vi "Stability Timer.vi"(0 "CommandCluster":T1, 2 "Mode":enum16{"Init", "Run"}(ring)=enum."Run", 7 "Stable":bool, 9 "Stable 2":bool, 11 "Stable 3":bool, 12 "time":refnum<vi>, 13 "time 2":refnum<vi>, 14 "time 3":refnum<vi>) -> (4 "GraphSig":bool, 15 "Stabilized?":bool)   [LabVIEW 2013]
uses:
  TypeDef/Command Cluster.ctl
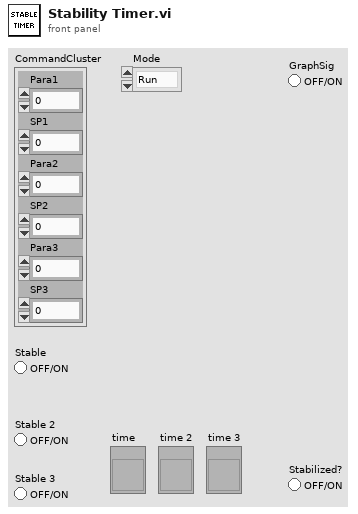
[diagram p1: front panel]
types:
  T1 = typedef "Command Cluster.ctl" = cluster{"Para1":i32, "SP1":dbl, "Para2":i32, "SP2":dbl, "Para3":i32, "SP3":dbl}
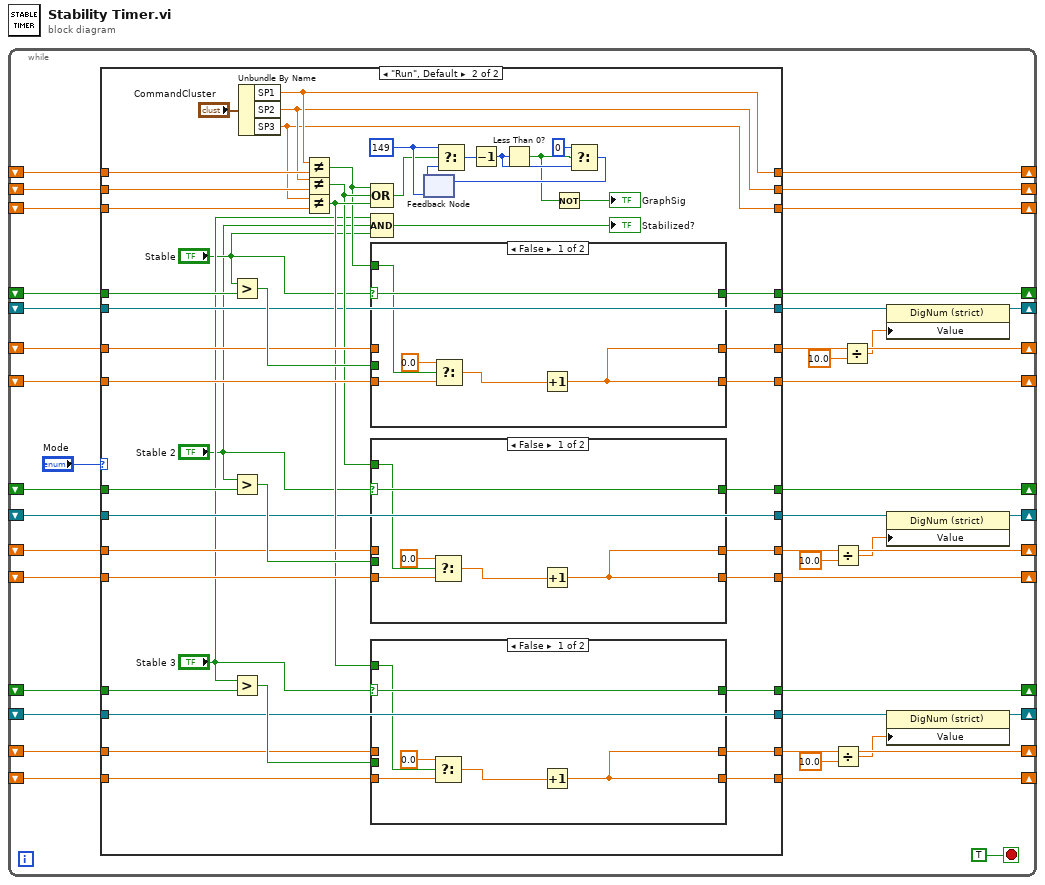
[diagram p0: block diagram]
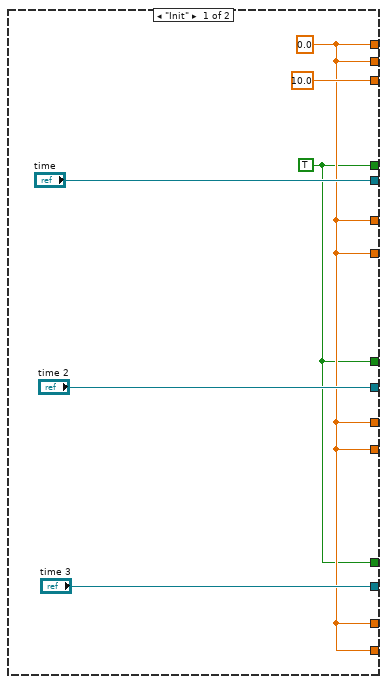
[diagram p2: hidden frame]
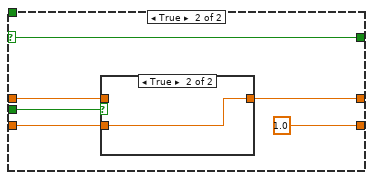
[diagram p3: hidden frame]
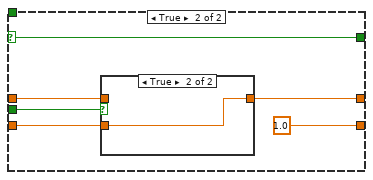
[diagram p5: hidden frame]
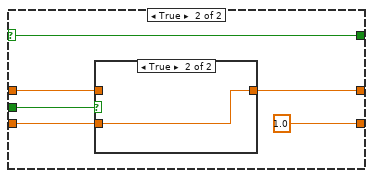
[diagram p7: hidden frame]
diagram:
  n1 = while {
    shift-right: [w40] -> _
    shift-left: _ -> [w37]
    shift-right: [w38] -> _
    shift-left: _ -> [w39]
    shift-right: [w36] -> _
    shift-left: _ -> [w35]
    shift-right: [w34] -> _
    shift-left: _ -> [w33]
    shift-right: [w10] -> _
    shift-left: _ -> [w32]
    shift-right: [w11] -> _
    shift-left: _ -> [w31]
    shift-right: [w28] -> _
    shift-left: _ -> [w29]
    shift-right: [w27] -> _
    shift-left: _ -> [w30]
    shift-right: [w26] -> _
    shift-left: _ -> [w21]
    shift-right: [w12] -> _
    shift-left: _ -> [w22]
    shift-right: [w25] -> _
    shift-left: _ -> [w20]
    shift-right: [w23] -> _
    shift-left: _ -> [w24]
    shift-right: [w5] -> _
    shift-left: _ -> [w16]
    shift-right: [w4] -> _
    shift-left: _ -> [w17]
    shift-right: [w8] -> _
    shift-left: _ -> [w18]
    stop <- TRUE stop-if-true
    n2 = case shown="\"Run\", Default" "Mode" {
      tunnel: [w42 w94] -> w40
      tunnel: w39 -> [_ w93]
      tunnel: [w43 w92] -> w38
      tunnel: w37 -> [_ w91]
      tunnel: [w42 w88] -> w36
      tunnel: w35 -> [_ w87]
      tunnel: [w43 w86] -> w34
      tunnel: w33 -> [_ w85]
      tunnel: [w43 w84] -> w10
      tunnel: w32 -> [_ w83]
      tunnel: [w43 w82] -> w11
      tunnel: w31 -> [_ w81]
      tunnel: w30 -> [_ w79]
      tunnel: w29 -> [_ w78]
      tunnel: [w43 w77] -> w28
      tunnel: [w43 w76] -> w27
      tunnel: [w43 w75] -> w12
      tunnel: [w43 w74] -> w26
      tunnel: [w42 w73] -> w25
      tunnel: w24 -> [_ w72]
      tunnel: [10.0 ("SP3") w71] -> w23
      tunnel: w22 -> [_ w69]
      tunnel: w21 -> [_ w68]
      tunnel: w20 -> [_ w67]
      tunnel: ["time" w63] -> w9
      tunnel: ["time 2" w62] -> w6
      tunnel: ["time 3" w61] -> w7
      tunnel: w18 -> [_ w63]
      tunnel: w17 -> [_ w62]
      tunnel: w16 -> [_ w61]
      frame "Init" {
        w42 = TRUE
        w43 = 0.0 ("SP1")
      }
      frame "Run", Default {
        w55 = 149
        n3 = Greater?(x="Stable", y=w91) -> (0:w90:bool)
        n4 = Greater?(x="Stable 2", y=w87) -> (0:w89:bool)
        n5 = Greater?(x="Stable 3", y=w67) -> (0:w70:bool)
        n6 = Unbundle By Name("CommandCluster") -> ("SP1"=w77:dbl, "SP2"=w76:dbl, "SP3"=w71:dbl)
        n7 = Not Equal?(x=w77, y=w78) -> (x != y?=w64:bool)
        n8 = Not Equal?(x=w76, y=w79) -> (x != y?=w65:bool)
        n9 = Not Equal?(x=w71, y=w72) -> (x != y?=w66:bool)
        n10 = Compound Arithmetic op=OR(w64, w65, w66) -> (w54:bool)
        n11 = Compound Arithmetic op=AND("Stable 3", "Stable 2", "Stable") -> (→"Stabilized?":bool)
        n12 = case shown="False" "Stable" {
          selector: "Stable" -> [w128 w133]
          tunnel: [w128 w133] -> w94
          tunnel: w93 -> [w125 w131]
          tunnel: [w127 1.0 ("y")] -> w92
          tunnel: w90 -> [_ w132]
          tunnel: [w127 w130] -> w84
          tunnel: w83 -> [_ w129]
          tunnel: w64 -> [w126 _]
          frame False {
            n13 = Select(t=0.0, s=w126, f=w125) -> (s? t:f=w124:dbl)
            n14 = Increment(x=w124) -> (x+1=w127:dbl)
          }
          frame True {
            n15 = case shown="True" w132 {
              tunnel: w131 -> [_ w136]
              tunnel: [w135 w136] -> w130
              tunnel: w129 -> [w135 _]
              frame False {
              }
              frame True {
              }
            }
          }
        }
        n16 = case shown="False" "Stable 2" {
          selector: "Stable 2" -> [w114 w119]
          tunnel: [w114 w119] -> w88
          tunnel: w85 -> [w111 w117]
          tunnel: [w113 1.0 ("y")] -> w86
          tunnel: w89 -> [_ w118]
          tunnel: [w113 w116] -> w82
          tunnel: w81 -> [_ w115]
          tunnel: w65 -> [w112 _]
          frame False {
            n17 = Select(t=0.0, s=w112, f=w111) -> (s? t:f=w110:dbl)
            n18 = Increment(x=w110) -> (x+1=w113:dbl)
          }
          frame True {
            n19 = case shown="True" w118 {
              tunnel: w117 -> [_ w122]
              tunnel: [w121 w122] -> w116
              tunnel: w115 -> [w121 _]
              frame False {
              }
              frame True {
              }
            }
          }
        }
        n20 = case shown="False" "Stable 3" {
          selector: "Stable 3" -> [w100 w105]
          tunnel: [w100 w105] -> w73
          tunnel: w68 -> [w97 w103]
          tunnel: [w99 1.0 ("y")] -> w74
          tunnel: w70 -> [_ w104]
          tunnel: [w99 w102] -> w75
          tunnel: w69 -> [_ w101]
          tunnel: w66 -> [w98 _]
          frame False {
            n21 = Select(t=0.0, s=w98, f=w97) -> (s? t:f=w96:dbl)
            n22 = Increment(x=w96) -> (x+1=w99:dbl)
          }
          frame True {
            n23 = case shown="True" w104 {
              tunnel: w103 -> [_ w108]
              tunnel: [w107 w108] -> w102
              tunnel: w101 -> [w107 _]
              frame False {
              }
              frame True {
              }
            }
          }
        }
        n24 = feedback #1(w55) -> (w56:i32)
        n25 = Select(t=w55, s=w54, f=w56) -> (s? t:f=w60:i32)
        n26 = Decrement(x=w60) -> (x-1=w59:i32)
        n27 = Less Than 0?(x=w59) -> (x < 0?=w53:bool)
        n28 = Not(x=w53) -> (.not. x?=→"GraphSig":bool)
        n29 = Select(t=0, s=w53, f=w59) -> (s? t:f=w57:i32)
        n30 = feedback-in #1(w57) -> ()
      }
    }
    n31 = Divide(x=w11, y=10.0) -> (x/y=w2:dbl)
    n32 = Divide(x=w12, y=10.0) -> (x/y=w3:dbl)
    n33 = Divide(x=w10, y=10.0) -> (x/y=w1:dbl)
    n34 = property class="DigNum (strict)"(reference=w9, "Value"=w1) -> (reference out=w8:refnum<vi>)  [unwired: 1 in, 1 out]
    n35 = property class="DigNum (strict)"(reference=w6, "Value"=w2) -> (reference out=w4:refnum<vi>)  [unwired: 1 in, 1 out]
    n36 = property class="DigNum (strict)"(reference=w7, "Value"=w3) -> (reference out=w5:refnum<vi>)  [unwired: 1 in, 1 out]
  }
